vi "Iso15765.vi"(4 "TransmittId":u32 format="%08x", 5 "BS":u8 format="%02x", 6 "ReceiveId":u32 format="%08x", 7 "STmin":u8 format="%02x", 8 "error in (no error)":errorcluster, 9 "TimeoutMs":u32, 10 "Request":u8[](array[numeric]) format="%02x", 11 "GenericCanAdapterClass in":refnum<class "GenericCanAdapterClass.lvclass">) -> (0 "error out":errorcluster, 2 "Response":u8[](array[numeric]) format="%02x", 3 "GenericCanAdapterClass out":refnum<class "GenericCanAdapterClass.lvclass">)   [LabVIEW 2011, in "GenericCanAdapterClass.lvclass"]
uses:
  GenericCanAdapterClass.lvclass
  Iso15765State_Type.ctl
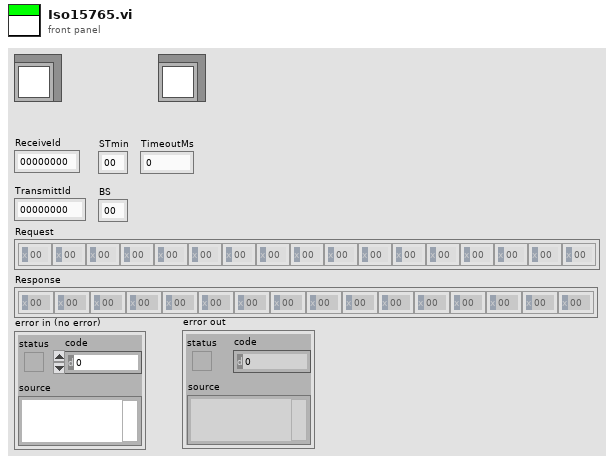
[diagram p1: front panel]
types:
  T1 = typedef "GenericCanAdapterClass.lvclass/Iso15765State_Type.ctl" = enum16{"ST_START", "ST_IDLE", "ST_TX_ERROR", "ST_TX", "ST_TX_SINGLE", "ST_TX_FIRST", "ST_RX_FLOWCTRL", "ST_TX_WAIT", "ST_TX_CONSECUTIVE", "ST_RX_ERROR", "ST_RX", "ST_TX_FLOWCTRL", "ST_RX_CONSECUTIVE", "ST_RX_DONE", "ST_RX_NOT_HANDLED_NRC", "ST_RETRY", "ST_COMPLETE"}
  T2 = typedef "GenericCanAdapterClass.lvclass/MessageType.ctl" = cluster{"Arbitration Id":u32, "Data":u8[], "DataLength":u16, "TimeStamp":timestamp}
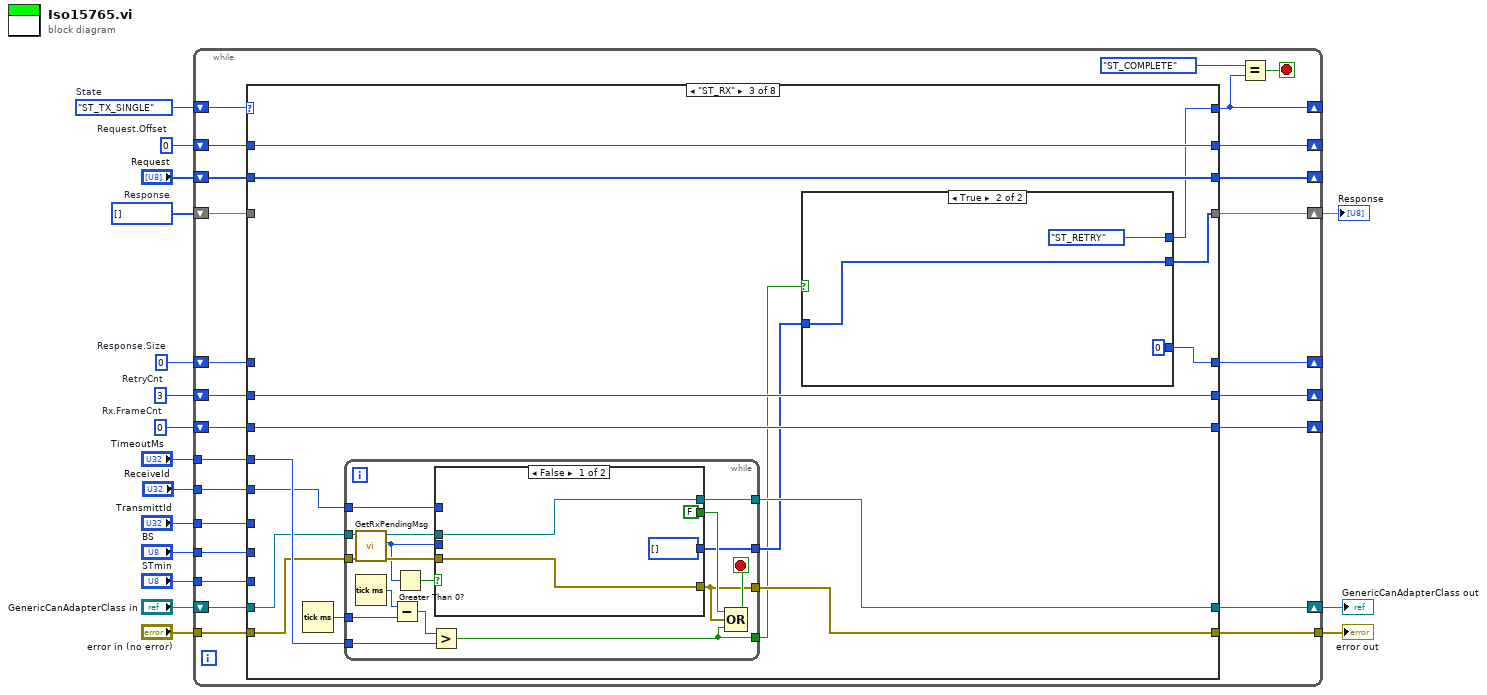
[diagram p0: block diagram]
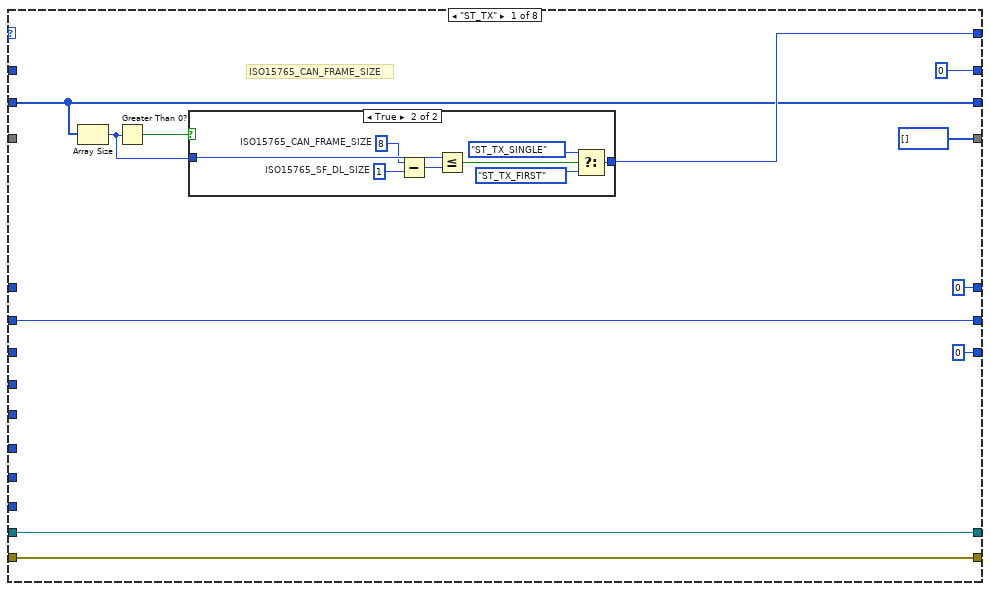
[diagram p2: hidden frame]
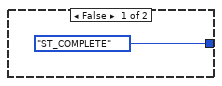
[diagram p3: hidden frame]
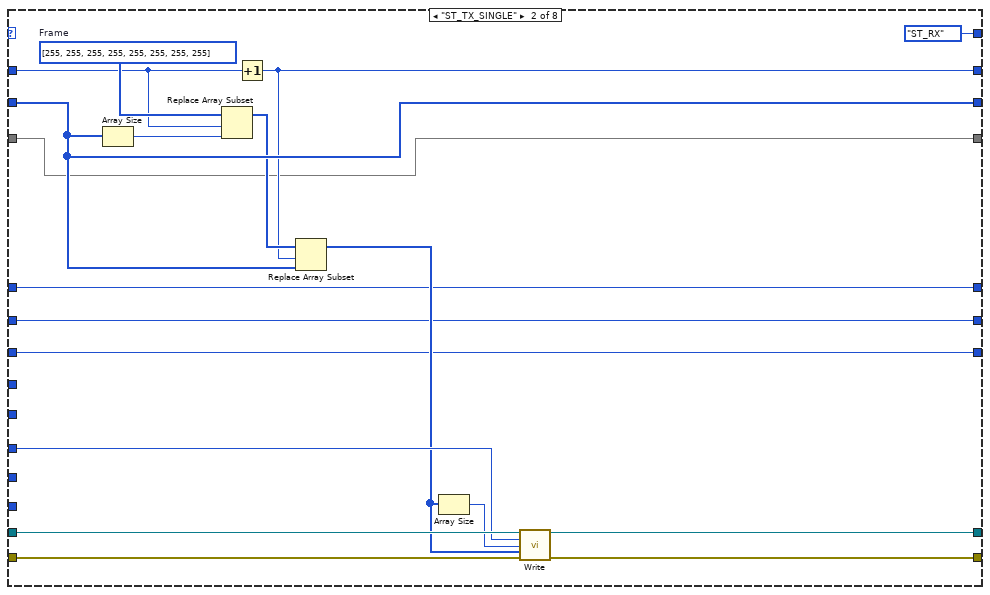
[diagram p4: hidden frame]
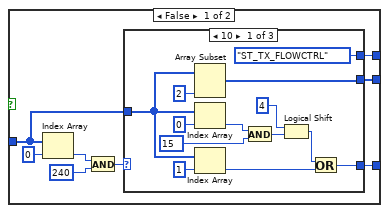
[diagram p5: hidden frame]
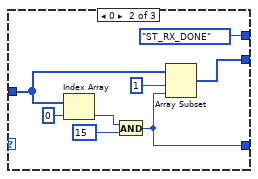
[diagram p6: hidden frame]
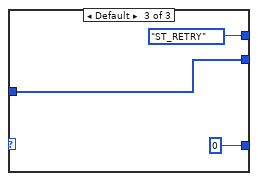
[diagram p7: hidden frame]
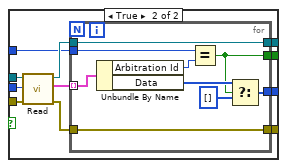
[diagram p8: hidden frame]
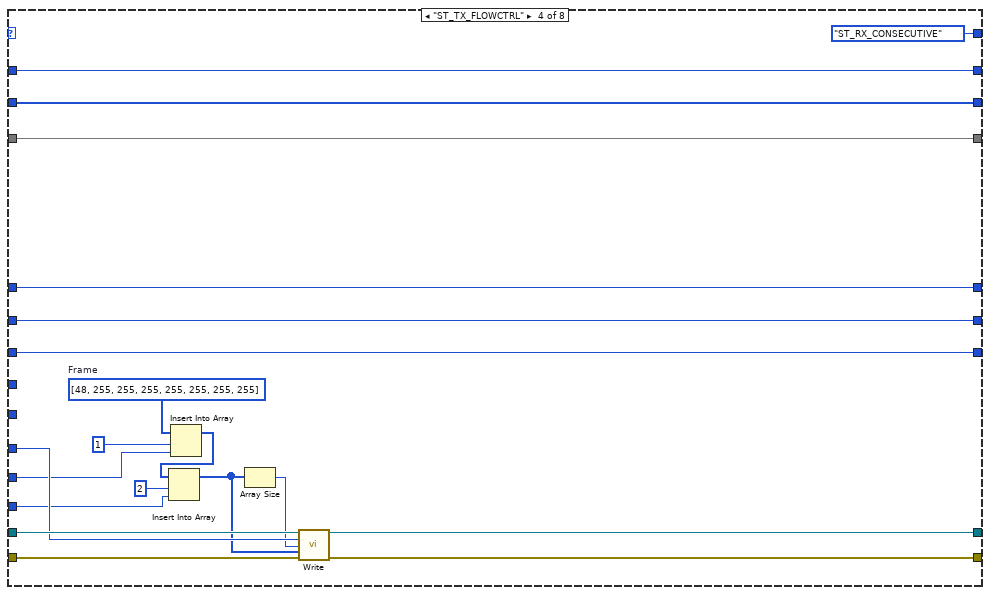
[diagram p9: hidden frame]
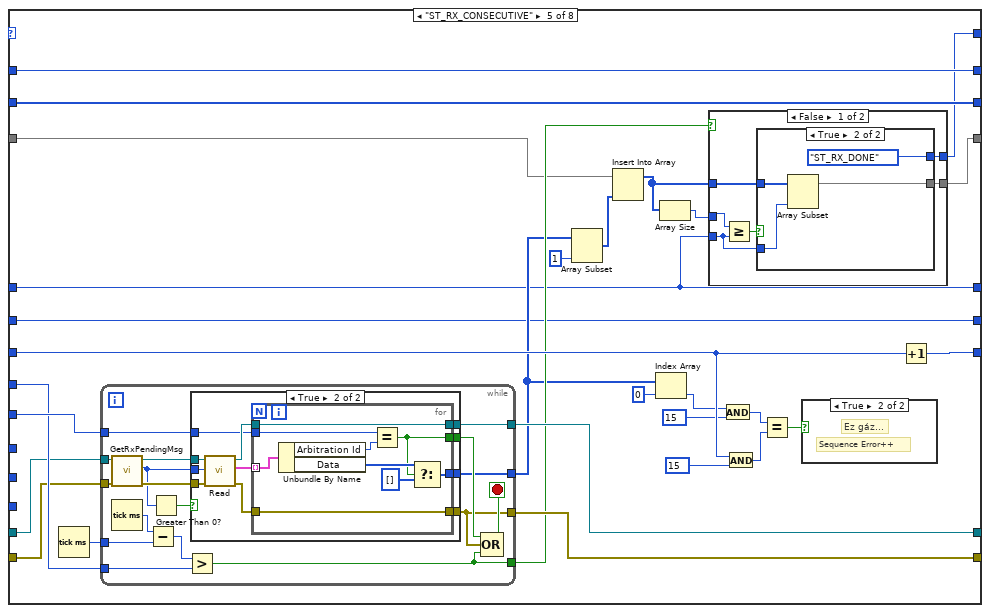
[diagram p10: hidden frame]
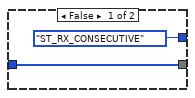
[diagram p11: hidden frame]
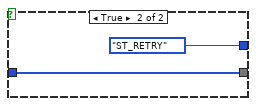
[diagram p12: hidden frame]
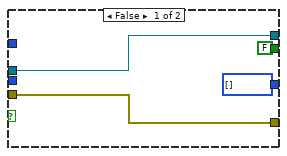
[diagram p14: hidden frame]
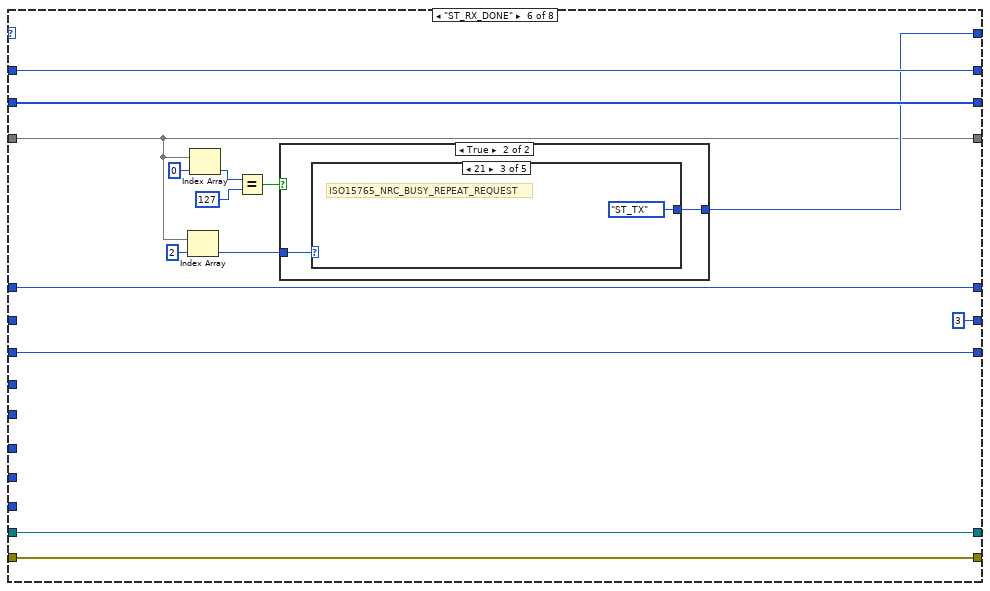
[diagram p15: hidden frame]
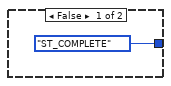
[diagram p16: hidden frame]
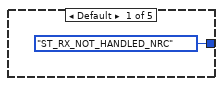
[diagram p17: hidden frame]
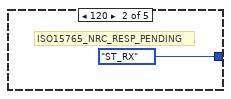
[diagram p18: hidden frame]
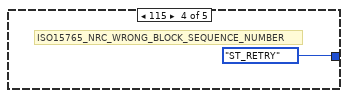
[diagram p19: hidden frame]
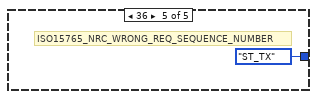
[diagram p20: hidden frame]
diagram:
  w1 = u16 3  # RetryCnt
  w2 = u8 0  # Rx.FrameCnt
  w8 = u16 0  # Response.Size
  w10 = u8[] []  # Response
  w12 = u32 0  # Request.Offset
  w15 = Iso15765State_Type."ST_TX_SINGLE"  # State
  n1 = while {
    tunnel: "error in (no error)" -> [w42]
    tunnel: [w41] -> w16
    shift-right: [w33] -> _
    shift-left: w15 -> [w40]
    shift-right: [w35] -> _
    shift-left: w12 -> [w37]
    shift-right: [w30] -> _
    shift-left: "Request" -> [w36]
    shift-right: [w31] -> w9
    shift-left: w10 -> [w32]
    shift-right: [w28] -> _
    shift-left: w8 -> [w29]
    tunnel: "TransmittId" -> [w27]
    tunnel: "BS" -> [w26]
    tunnel: "STmin" -> [w25]
    tunnel: "ReceiveId" -> [w24]
    tunnel: "TimeoutMs" -> [w23]
    shift-right: [w21] -> _
    shift-left: w2 -> [w22]
    shift-right: [w19] -> _
    shift-left: w1 -> [w20]
    shift-right: [w39] -> w13
    shift-left: "GenericCanAdapterClass in" -> [w38]
    stop <- w18 stop-if-true
    n2 = case shown="\"ST_RX\"" w40 {
      selector: w40 -> [_ _ _ _ _ _ w307 _]
      tunnel: [w53 w79 w83 w191 w215 w285 w308 w309] -> w41
      tunnel: w42 -> [w53 w80 w87 w192 w216 w285 w308 w310]
      tunnel: [w49 Iso15765State_Type."ST_RX" ("Iso15765State_Type") w92 Iso15765State_Type."ST_RX_CONSECUTIVE" w205 w280 w307 w311] -> w33
      tunnel: [w52 w78 w84 w190 w214 w286 w306 w318] -> w39
      tunnel: w38 -> [w52 w77 w86 w189 w199 w286 w306 w318]
      tunnel: w37 -> [_ w73 w95 w176 w221 w291 _ w314]
      tunnel: w36 -> [w46 w71 w96 w177 w220 w290 w303 w315]
      tunnel: [u32 0 ("Request.Offset") w67 w95 w176 w221 w291 u32 0 ("Request.Offset") w314] -> w35
      tunnel: [u8[] [] ("Request") w65 w91 w178 w194 w278 w304 w316] -> w31
      tunnel: w32 -> [_ w65 _ w178 w204 w278 w304 w316]
      tunnel: [w46 w71 w96 w177 w220 w290 w303 w315] -> w30
      tunnel: w29 -> [_ w64 _ w179 w196 w288 w302 w317]
      tunnel: [u16 0 ("Response.Size") w64 w93 w179 w196 w288 w302 w317] -> w28
      tunnel: w27 -> [_ w70 _ w188 _ _ _ _]
      tunnel: w26 -> [_ _ _ w184 _ _ _ _]
      tunnel: w25 -> [_ _ _ w183 _ _ _ _]
      tunnel: w24 -> [_ _ w85 _ w218 _ _ _]
      tunnel: w23 -> [_ _ w88 _ w217 _ _ _]
      tunnel: [u8 0 ("Rx.FrameCnt") w63 w94 w174 w213 w287 w301 w319] -> w21
      tunnel: w22 -> [_ w63 w94 w174 w211 w287 w301 w319]
      tunnel: w20 -> [w43 w66 w90 w173 w193 _ w300 w320]
      tunnel: [w43 w66 w90 w173 w193 u16 3 ("RetryCnt") w300 w312] -> w19
      frame "ST_TX" {
        # "ISO15765_CAN_FRAME_SIZE"
        n3 = Array Size(array=w46) -> (size(s)=w47:i32)
        n4 = Greater Than 0?(x=w47) -> (x > 0?=w51:bool)
        n5 = case shown="True" w51 {
          tunnel: w47 -> [_ w58]
          tunnel: [Iso15765State_Type."ST_COMPLETE" ("Iso15765State_Type") w57] -> w49
          frame False {
          }
          frame True {
            w55 = 1  # ISO15765_SF_DL_SIZE
            w56 = 8  # ISO15765_CAN_FRAME_SIZE
            n6 = Subtract(x=w56, y=w55) -> (x-y=w62:i32)
            n7 = Less Or Equal?(x=w58, y=w62) -> (x <= y?=w61:bool)
            n8 = Select(t=Iso15765State_Type."ST_TX_SINGLE" ("Iso15765State_Type"), s=w61, f=Iso15765State_Type."ST_TX_FIRST" ("Iso15765State_Type")) -> (s? t:f=w57:T1)
          }
        }
      }
      frame "ST_TX_SINGLE" {
        w76 = u8[] [255, 255, 255, 255, 255, 255, 255, 255]  # Frame
        n9 = Array Size(array=w71) -> (size(s)=w72:i32)
        n10 = Replace Array Subset(array=w76, new element=w72, index=w73) -> (w69:u8[])
        n11 = Increment(x=w73) -> (x+1=w67:u32)
        n12 = Replace Array Subset(array=w69, new element=w71, index=w67) -> (w68:u8[])
        n13 = Array Size(array=w68) -> (size(s)=w75:i32)
        n14 = call-dynamic "Write.vi"("GenericCanAdapterClass in"=w77, "Id"=w70, "DataLength"=w75, "Data"=w68, "error in (no error)"=w80) -> ("GenericCanAdapterClass out"=w78:refnum<class "GenericCanAdapterClass.lvclass">, "error out"=w79:errorcluster)  [unwired: 9 in]
      }
      frame "ST_RX" {
        n15 = Tick Count (ms)() -> (millisecond timer value=w89:u32)
        n16 = while {
          tunnel: [w136] -> w83
          tunnel: [w147] -> w84
          tunnel: w85 -> [w143]
          tunnel: w89 -> [w141]
          tunnel: w88 -> [w138]
          tunnel: [w135] -> w82
          tunnel: w87 -> [w134]
          tunnel: w86 -> [w133]
          tunnel: [w132] -> w81
          stop <- w142 stop-if-true
          n17 = call-dynamic "GetRxPendingMsg.vi"("error in (no error)"=w134, "GenericCanAdapterClass in"=w133) -> ("error out"=w148:errorcluster, "Value"=w144:i32, "GenericCanAdapterClass out"=w146:refnum<class "GenericCanAdapterClass.lvclass">)  [unwired: 7 in]
          n18 = Tick Count (ms)() -> (millisecond timer value=w140:u32)
          n19 = Subtract(x=w140, y=w141) -> (x-y=w139:u32)
          n20 = Greater Than 0?(x=w144) -> (x > 0?=w145:bool)
          n21 = Greater?(x=w139, y=w138) -> (0:w132:bool)
          n22 = case shown="False" w145 {
            tunnel: w148 -> [w151 w163]
            tunnel: [w151 w157] -> w136
            tunnel: [w152 w159] -> w147
            tunnel: w146 -> [w152 w162]
            tunnel: w144 -> [_ w161]
            tunnel: w143 -> [_ w155]
            tunnel: [FALSE w154] -> w137
            tunnel: [u8[] [] ("f") w153] -> w135
            frame False {
            }
            frame True {
              n23 = call "Read.vi"("error in (no error)"=w163, "Request Number of Message"=w161, "GenericCanAdapterClass in"=w162) -> ("error out"=w156:errorcluster, "Messages"=w160:T2[], "GenericCanAdapterClass out"=w158:refnum<class "GenericCanAdapterClass.lvclass">)  [unwired: 6 in]
              n24 = for {
                tunnel: w160 -> [w170] mode=indexing
                tunnel: [w172] -> w159
                tunnel: w158 -> [w172]
                tunnel: [w171] -> w157
                tunnel: w156 -> [w171]
                tunnel: w155 -> [w169]
                tunnel: [w166] -> w154
                tunnel: [w164] -> w153
                n25 = Unbundle By Name(w170) -> ("Arbitration Id"=w168:u32, "Data"=w167:u8[])
                n26 = Equal?(x=w169, y=w168) -> (x = y?=w166:bool)
                n27 = Select(t=w167, s=w166, f=u8[] []) -> (s? t:f=w164:u8[])
              }
            }
          }
          n28 = Compound Arithmetic op=OR(w137, w136, w132) -> (w142:bool)
        }
        n29 = case shown="True" w81 {
          tunnel: [w100 u8 0] -> w93
          tunnel: [w99 Iso15765State_Type."ST_RETRY" ("Iso15765State_Type")] -> w92
          tunnel: [w98 w129] -> w91
          tunnel: w82 -> [w97 w129]
          frame False {
            n30 = Index Array(array=w97, index=0) -> (element=w101:u8)
            n31 = And(x=w101, y=u8 240) -> (x .and. y?=w103:u8)
            n32 = case shown="10" w103 {
              tunnel: [Iso15765State_Type."ST_TX_FLOWCTRL" ("f") Iso15765State_Type."ST_RX_DONE" ("Iso15765State_Type") Iso15765State_Type."ST_RETRY" ("Iso15765State_Type")] -> w99
              tunnel: w97 -> [w107 w120 w126]
              tunnel: [w106 w119 w126] -> w98
              tunnel: [w105 w118 u8 0] -> w100
              frame 16 {
                n33 = Array Subset(array=w107, length=2) -> (w106:u8[])  [unwired: 1 in]
                n34 = Index Array(array=w107, index=0) -> (element=w109:u8)
                n35 = Index Array(array=w107, index=1) -> (element=w115:u8)
                n36 = And(x=w109, y=u8 15) -> (x .and. y?=w112:u8)
                n37 = Logical Shift(y=i8 4, x=w112) -> (x << y=w114:u8)
                n38 = Or(x=w114, y=w115) -> (x .or. y?=w105:u8)
              }
              frame 0 {
                n39 = Index Array(array=w120, index=0) -> (element=w122:u8)
                n40 = And(x=w122, y=u8 15) -> (x .and. y?=w118:u8)
                n41 = Array Subset(array=w120, index=1, length=w118) -> (w119:u8[])
              }
              frame Default {
              }
            }
          }
          frame True {
          }
        }
      }
      frame "ST_TX_FLOWCTRL" {
        w187 = u8[] [48, 255, 255, 255, 255, 255, 255, 255]  # Frame
        n42 = Insert Into Array(array=w187, index=1, new element=w184) -> (w185:u8[])
        n43 = Insert Into Array(array=w185, index=2, new element=w183) -> (w181:u8[])
        n44 = Array Size(array=w181) -> (size(s)=w180:i32)
        n45 = call-dynamic "Write.vi"("GenericCanAdapterClass in"=w189, "Id"=w188, "DataLength"=w180, "Data"=w181, "error in (no error)"=w192) -> ("GenericCanAdapterClass out"=w190:refnum<class "GenericCanAdapterClass.lvclass">, "error out"=w191:errorcluster)  [unwired: 9 in]
      }
      frame "ST_RX_CONSECUTIVE" {
        n46 = Tick Count (ms)() -> (millisecond timer value=w219:u32)
        n47 = while {
          tunnel: [w240] -> w215
          tunnel: [w251] -> w214
          tunnel: w218 -> [w247]
          tunnel: w219 -> [w245]
          tunnel: w217 -> [w242]
          tunnel: [w239] -> w203
          tunnel: w216 -> [w238]
          tunnel: w199 -> [w237]
          tunnel: [w236] -> w206
          stop <- w246 stop-if-true
          n48 = call-dynamic "GetRxPendingMsg.vi"("error in (no error)"=w238, "GenericCanAdapterClass in"=w237) -> ("error out"=w252:errorcluster, "Value"=w248:i32, "GenericCanAdapterClass out"=w250:refnum<class "GenericCanAdapterClass.lvclass">)  [unwired: 7 in]
          n49 = Tick Count (ms)() -> (millisecond timer value=w244:u32)
          n50 = Subtract(x=w244, y=w245) -> (x-y=w243:u32)
          n51 = Greater Than 0?(x=w248) -> (x > 0?=w249:bool)
          n52 = Greater?(x=w243, y=w242) -> (0:w236:bool)
          n53 = case shown="True" w249 {
            tunnel: w252 -> [w255 w267]
            tunnel: [w255 w261] -> w240
            tunnel: [w256 w263] -> w251
            tunnel: w250 -> [w256 w266]
            tunnel: w248 -> [_ w265]
            tunnel: w247 -> [_ w259]
            tunnel: [FALSE w258] -> w241
            tunnel: [u8[] [] ("f") w257] -> w239
            frame False {
            }
            frame True {
              n54 = call "Read.vi"("error in (no error)"=w267, "Request Number of Message"=w265, "GenericCanAdapterClass in"=w266) -> ("error out"=w260:errorcluster, "Messages"=w264:T2[], "GenericCanAdapterClass out"=w262:refnum<class "GenericCanAdapterClass.lvclass">)  [unwired: 6 in]
              n55 = for {
                tunnel: w264 -> [w274] mode=indexing
                tunnel: [w276] -> w263
                tunnel: w262 -> [w276]
                tunnel: [w275] -> w261
                tunnel: w260 -> [w275]
                tunnel: w259 -> [w273]
                tunnel: [w270] -> w258
                tunnel: [w268] -> w257
                n56 = Unbundle By Name(w274) -> ("Arbitration Id"=w272:u32, "Data"=w271:u8[])
                n57 = Equal?(x=w273, y=w272) -> (x = y?=w270:bool)
                n58 = Select(t=w271, s=w270, f=u8[] []) -> (s? t:f=w268:u8[])
              }
            }
          }
          n59 = Compound Arithmetic op=OR(w241, w240, w236) -> (w246:bool)
        }
        n60 = Array Subset(array=w203, length=1) -> (w198:u8[])  [unwired: 1 in]
        n61 = Insert Into Array(array=w204, new element=w198) -> (w195:u8[])  [unwired: 1 in]
        n62 = Index Array(array=w203, index=0) -> (element=w208:u8)
        n63 = Array Size(array=w195) -> (size(s)=w197:i32)
        n64 = case shown="False" w206 {
          tunnel: [w223 Iso15765State_Type."ST_RETRY"] -> w205
          tunnel: w197 -> [w226 _]
          tunnel: w196 -> [w222 _]
          tunnel: w195 -> [w225 w234]
          tunnel: [w224 w234] -> w194
          frame False {
            n65 = Greater Or Equal?(x=w226, y=w222) -> (x >= y?=w227:bool)
            n66 = case shown="True" w227 {
              tunnel: w222 -> [_ w232]
              tunnel: w225 -> [w228 w233]
              tunnel: [w228 w231] -> w224
              tunnel: [Iso15765State_Type."ST_RX_CONSECUTIVE" ("Iso15765State_Type") Iso15765State_Type."ST_RX_DONE" ("Iso15765State_Type")] -> w223
              frame False {
              }
              frame True {
                n67 = Array Subset(array=w233, length=w232) -> (w231:u8[])  [unwired: 1 in]
              }
            }
          }
          frame True {
          }
        }
        n68 = And(x=w208, y=u8 15) -> (x .and. y?=w200:u8)
        n69 = And(x=w211, y=u8 15) -> (x .and. y?=w201:u8)
        n70 = Equal?(x=w200, y=w201) -> (x = y?=w207:bool)
        n71 = case shown="True" w207 {
          frame False {
          }
          frame True {
            # "Sequence Error++"
            # "Ez gáz..."
          }
        }
        n72 = Increment(x=w211) -> (x+1=w213:u8)
      }
      frame "ST_RX_DONE" {
        n73 = Index Array(array=w278, index=2) -> (element=w277:u8)
        n74 = Index Array(array=w278, index=0) -> (element=w283:u8)
        n75 = Equal?(x=w283, y=u8 127) -> (x = y?=w281:bool)
        n76 = case shown="True" w281 {
          tunnel: [Iso15765State_Type."ST_COMPLETE" ("Iso15765State_Type") w293] -> w280
          tunnel: w277 -> [_ w294]
          frame False {
          }
          frame True {
            n77 = case shown="21" w294 {
              tunnel: [Iso15765State_Type."ST_RX_NOT_HANDLED_NRC" ("Iso15765State_Type") Iso15765State_Type."ST_RX" ("Iso15765State_Type") Iso15765State_Type."ST_TX" ("Iso15765State_Type") Iso15765State_Type."ST_RETRY" ("Iso15765State_Type") Iso15765State_Type."ST_TX" ("Iso15765State_Type")] -> w293
              frame Default {
              }
              frame 120 {
                # "ISO15765_NRC_RESP_PENDING"
              }
              frame 33 {
                # "ISO15765_NRC_BUSY_REPEAT_REQUEST"
              }
              frame 115 {
                # "ISO15765_NRC_WRONG_BLOCK_SEQUENCE_NUMBER"
              }
              frame 36 {
                # "ISO15765_NRC_WRONG_REQ_SEQUENCE_NUMBER"
              }
            }
          }
        }
      }
      frame "ST_IDLE", Default {
      }
      frame "ST_RETRY" {
        n78 = Decrement(x=w320) -> (x-1=w312:u16)
        n79 = Equal To 0?(x=w312) -> (x = 0?=w313:bool)
        n80 = case shown="True" w313 {
          tunnel: [Iso15765State_Type."ST_TX" ("Iso15765State_Type") Iso15765State_Type."ST_COMPLETE" ("Iso15765State_Type")] -> w311
          tunnel: w310 -> [w321 w324]
          tunnel: [w321 w323] -> w309
          frame False {
          }
          frame True {
            n81 = control-ref of="This VI"() -> (w326:refnum<vi>)
            n82 = call "ErrorHelper.vi"("Message"="Failed", "Code"=-8100 ("code"), "This VI"=w326) -> ("error out"=w325:errorcluster)
            n83 = Merge Errors(w325, w324) -> (w323:errorcluster)
          }
        }
      }
    }
    n84 = Equal?(x=Iso15765State_Type."ST_COMPLETE" ("Iso15765State_Type"), y=w33) -> (x = y?=w18:bool)
  }
  "GenericCanAdapterClass out" <- w13
  "error out" <- w16
  "Response" <- w9
